vi "IntegerSynByteArrayBulk.vi"(0 "Mode":T1(ring)=enum."Heterodyne", 7 "Input  F1 array":dbl[](array[numeric]), 8 "Clock multiplier":i32=64, 9 "Local Oscillator (IF,f2)":dbl, 10 "f (f1)":i32, 11 "Phase (degrees)":dbl=90.0) -> (3 "output array":u8[](array[numeric]) format="%08b")   [LabVIEW 2015]
panel:
  out "phase":u8 format="%08b"
  # "Heterodyne"
  # "IOtech      Synth           NatInstBrd\n              function          J7          P3                   P1\n              syn1 w clk       A0           3             P0.0  1\n              syn1 D7           A1           5             P0.1  3\n              syn2 w clk       A2           7             PO.2  5\n              syn2 D7           A3           9             PO.3  7\n              syn3 w clk       A4           4             PO.4  9\n              syn3 D7           A5           6             P0.5   11\n              syn1,2 FQ_UD  A6           8             PO.6   13\n              syn3 FQ_UD     A7          10            PO.7   15\n\n              Reset 1,2,3     B4          14             PFI3   23\n\n              SCLK              B0           13            PFI 0  17\n              SYNC              B1           15            PFI 1  19\n              DIN                B2           17             PFI 2  21"
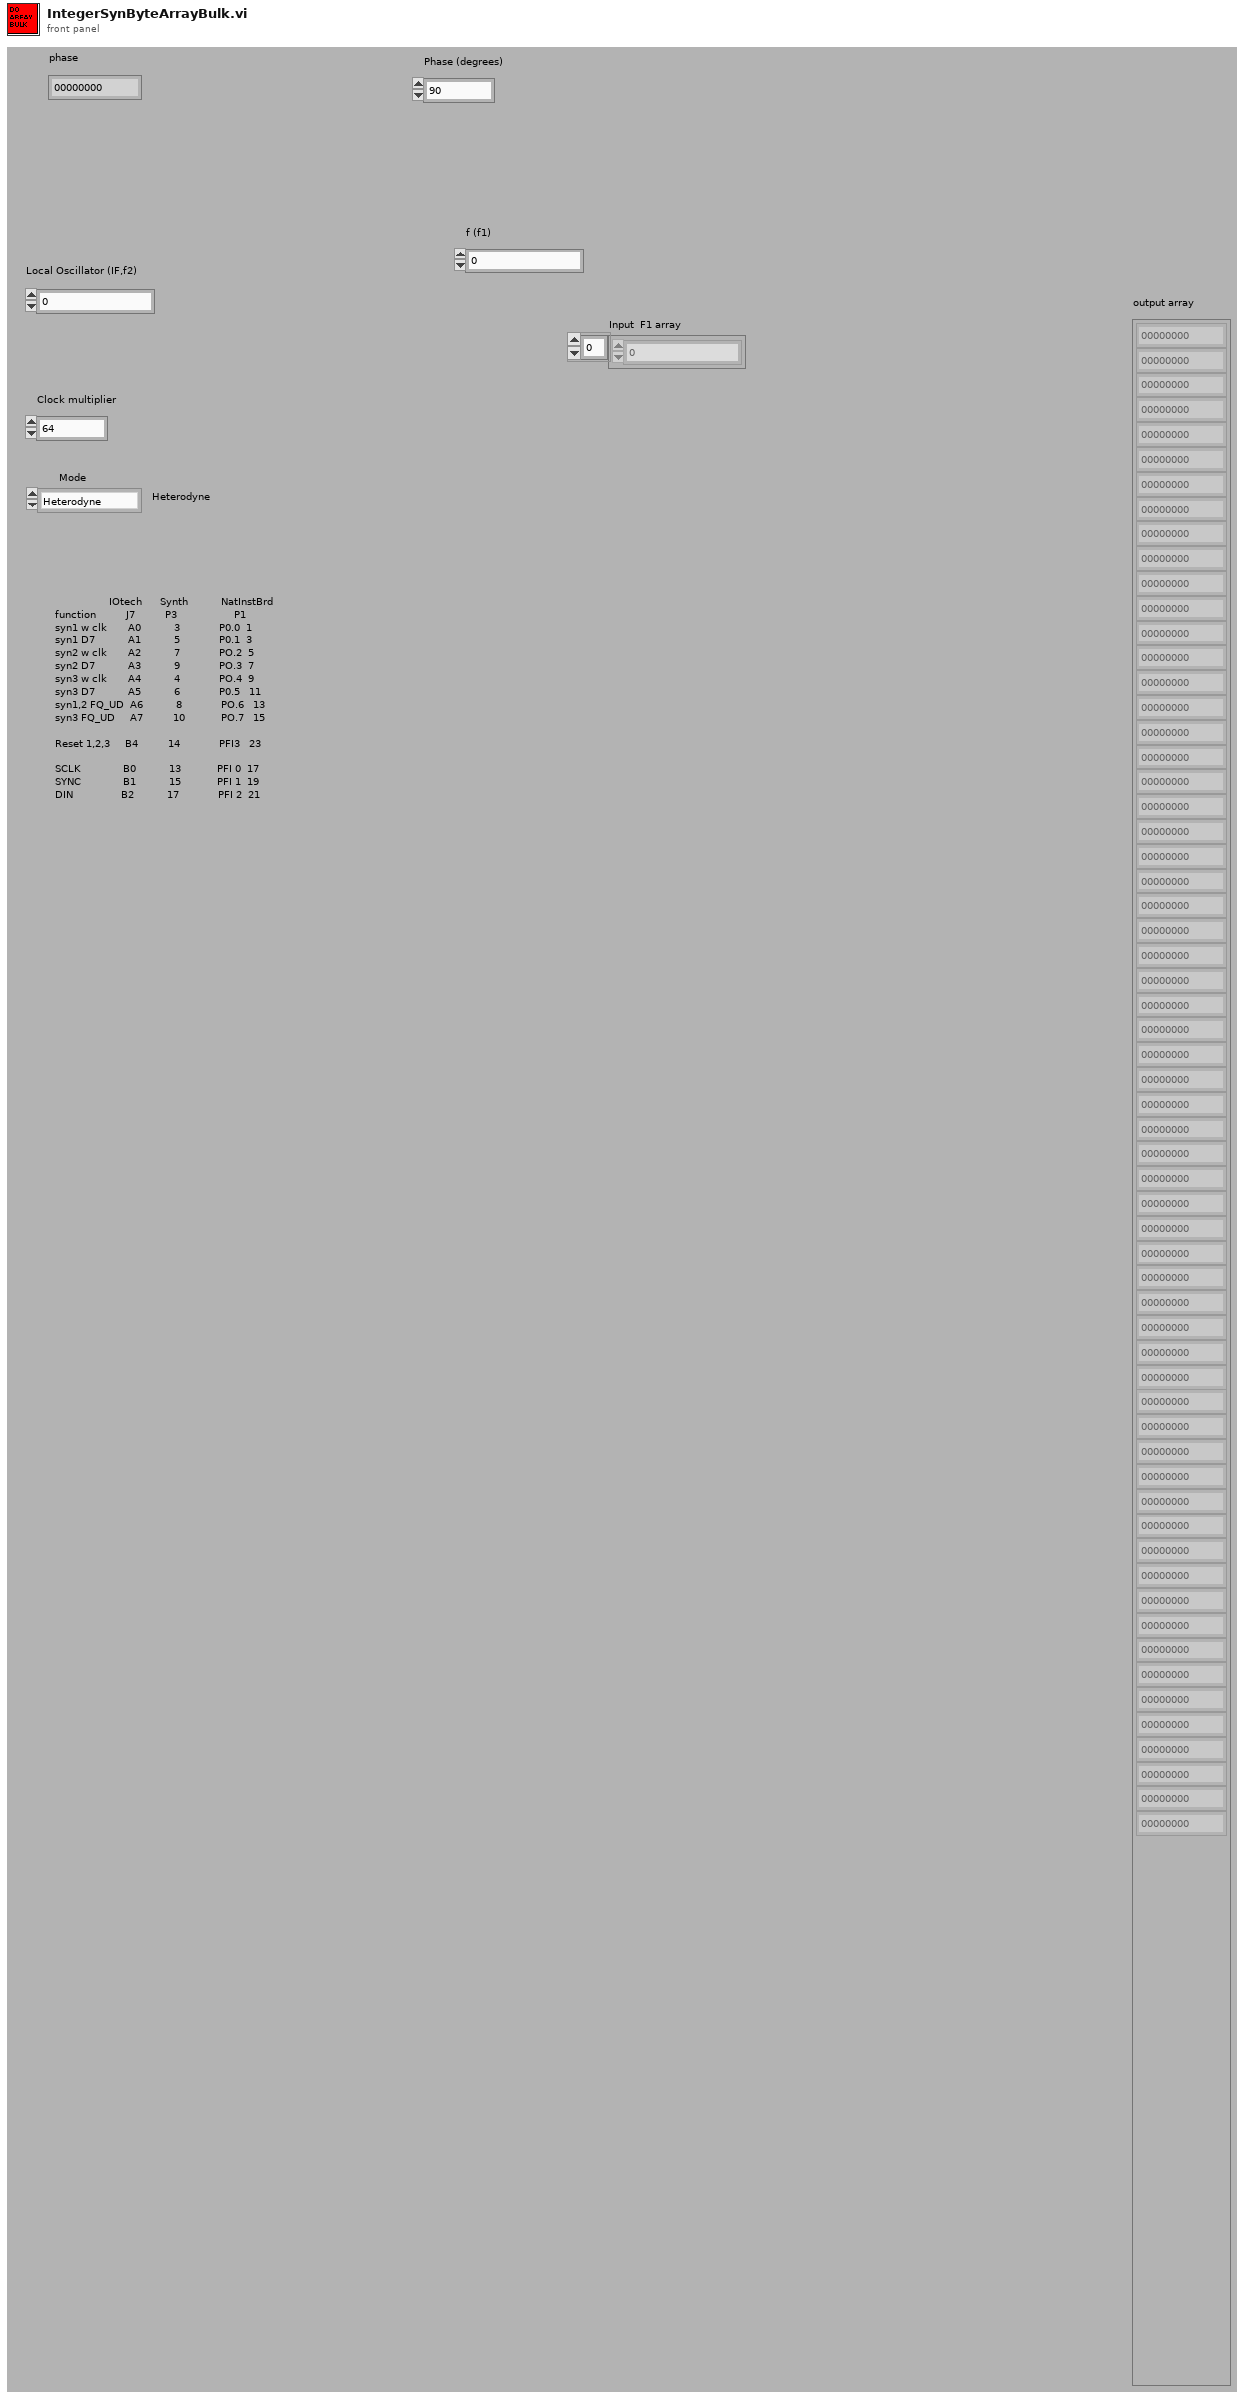
[diagram p1: front panel]
types:
  T1 = enum16{"Direct, clock*f1", "Direct, clock*f2", "Heterodyne"}
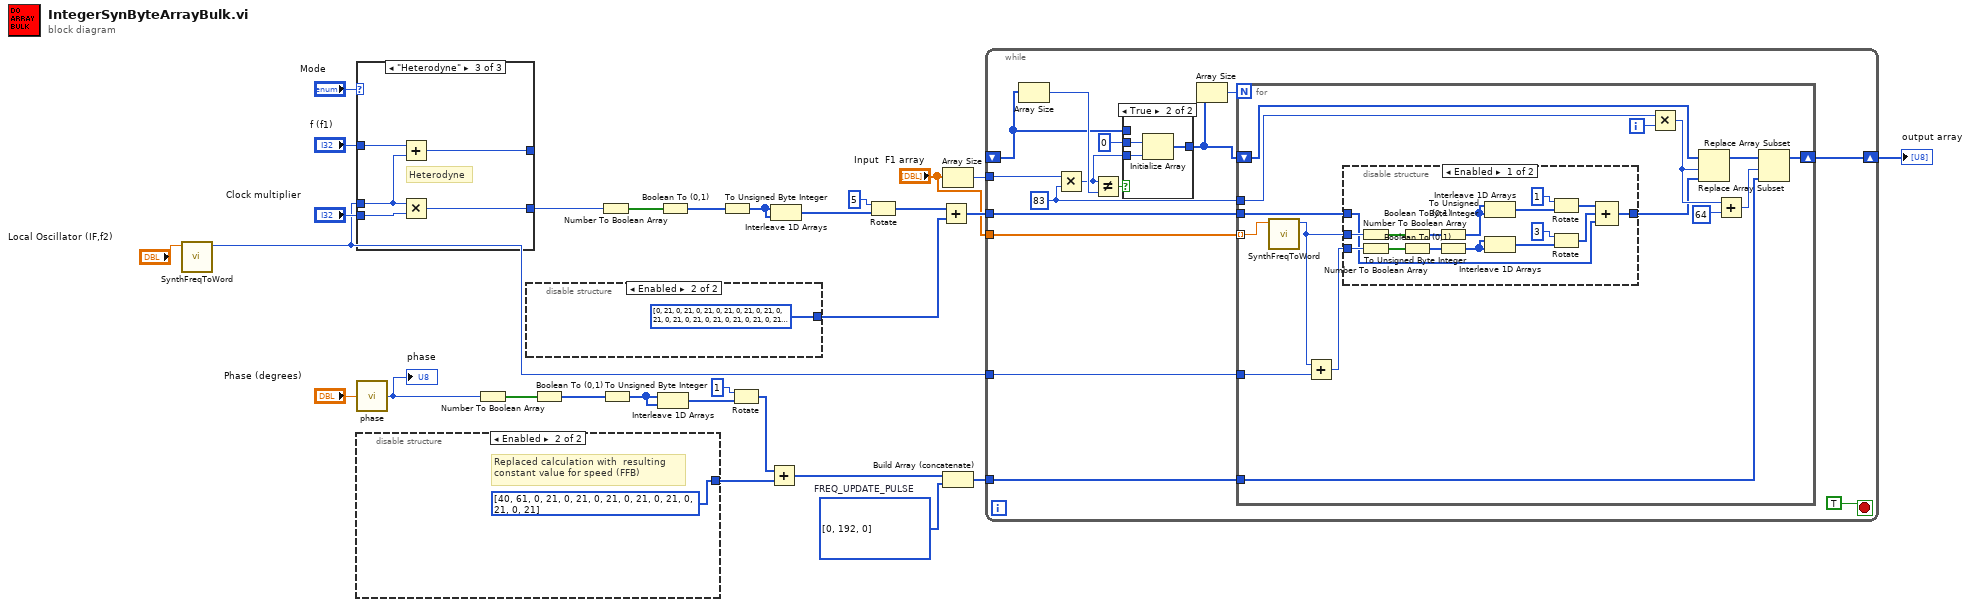
[diagram p0: block diagram]
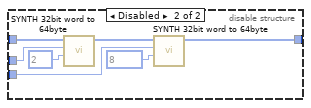
[diagram p3: hidden frame]
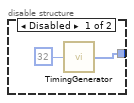
[diagram p4: hidden frame]
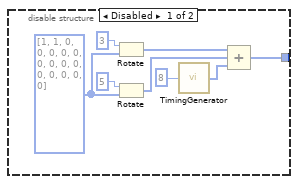
[diagram p5: hidden frame]
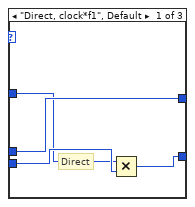
[diagram p6: hidden frame]
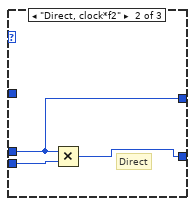
[diagram p7: hidden frame]
diagram:
  w3 = u8[] [0, 192, 0]  # FREQ_UPDATE_PULSE
  n1 = call "SynthFreqToWord.vi"("Frequency (Hz)"="Local Oscillator (IF,f2)") -> ("f-word out"=w5:u32)  [unwired: 8 in, 2 out]
  n2 = case shown="\"Heterodyne\"" "Mode" {
    tunnel: w5 -> [w31 w34 w39]
    tunnel: [w33 w36 w41] -> w24
    tunnel: "Clock multiplier" -> [w32 w35 w40]
    tunnel: [w31 w34 w37] -> _
    tunnel: "f (f1)" -> [w30 _ w38]
    frame "Direct, clock*f1", Default {
      # "Direct"
      n3 = Multiply(x=w30, y=w32) -> (x*y=w33:i32)
    }
    frame "Direct, clock*f2" {
      # "Direct"
      n4 = Multiply(x=w34, y=w35) -> (x*y=w36:u32)
    }
    frame "Heterodyne" {
      # "Heterodyne"
      n5 = Add(x=w38, y=w39) -> (x+y=w37:u32)
      n6 = Multiply(x=w39, y=w40) -> (x*y=w41:u32)
    }
  }
  n7 = call "phase.vi"("Phase"="Phase (degrees)") -> ("Phase Byte"=w18:u8)
  "phase" <- w18
  n8 = disable-structure shown="Enabled" {
    disable-tunnel: [w42 u8[] [40, 61, 0, 21, 0, 21, 0, 21, 0, 21, 0, 21, 0, 21, 0, 21] ("result")] -> w13
    frame Disabled {
      w44 = u8[] [1, 1, 0, 0, 0, 0, 0, 0, 0, 0, 0, 0, 0, 0, 0, 0] ("value")
      n9 = Rotate(1:w44, 2:i8 3) -> (0:w46:u8[])
      n10 = Rotate(1:w44, 2:i8 5) -> (0:w45:u8[])
      n11 = call "TimingGenerator.vi"("Clk String Lngth"=i8 8) -> ("TimingClock"=w43:u8[])
      n12 = Compound Arithmetic op=ADD(w46, w45, w43) -> (w42:u8[])
    }
    frame Enabled {
      # "Replaced calculation with  resulting \nconstant value for speed (FFB)"
    }
  }
  n13 = Number To Boolean Array(number=w18) -> (Boolean array=w21:bool[])
  n14 = disable-structure shown="Enabled" {
    disable-tunnel: [w51 u8[] [0, 21, 0, 21, 0, 21, 0, 21, 0, 21, 0, 21, 0, 21, 0, 21, 0, 21, 0, 21, 0, 21, 0, 21, 0, 21, 0, 21, 0, 21, 0, 21, 0, 21, 0, 21, 0, 21, 0, 21, 0, 21, 0, 21, 0, 21, 0, 21, 0, 21, 0, 21, 0, 21, 0, 21, 0, 21, 0, 21, 0, 21, 0, 21] ("TimingClock")] -> w7
    frame Disabled {
      n15 = call "TimingGenerator.vi"("Clk String Lngth"=i8 32) -> ("TimingClock"=w51:u8[])
    }
    frame Enabled {
    }
  }
  n16 = Boolean To (0,1)(Boolean=w21) -> (0, 1=w20:i16[])
  n17 = Number To Boolean Array(number=w24) -> (Boolean array=w28:bool[])
  n18 = To Unsigned Byte Integer(number=w20) -> (unsigned 8bit integer=w17:u8[])
  n19 = Interleave 1D Arrays(w17, w17) -> (w19:u8[])
  n20 = Boolean To (0,1)(Boolean=w28) -> (0, 1=w27:i16[])
  n21 = To Unsigned Byte Integer(number=w27) -> (unsigned 8bit integer=w22:u8[])
  n22 = Rotate(1:w19, 2:1) -> (0:w12:u8[])
  n23 = Add(x=w12, y=w13) -> (x+y=w9:u8[])
  n24 = Interleave 1D Arrays(w22, w22) -> (w26:u8[])
  n25 = Rotate(1:w26, 2:i8 5) -> (0:w11:u8[])
  n26 = Add(x=w11, y=w7) -> (x+y=w10:u8[])
  n27 = Array Size(array="Input  F1 array") -> (size(s)=w2:i32)
  n28 = Build Array (concatenate)(w9, w3) -> (w4:u8[])
  n29 = while {
    tunnel: w10 -> [w68]
    tunnel: w5 -> [w66]
    tunnel: w4 -> [w65]
    shift-right: [w67] -> w8
    shift-left: _ -> [w58]
    tunnel: w2 -> [w64]
    tunnel: "Input  F1 array" -> [w57]
    stop <- TRUE stop-if-true
    w63 = 83
    n30 = Array Size(array=w58) -> (size(s)=w62:i32)
    n31 = Multiply(x=w64, y=w63) -> (x*y=w60:i32)
    n32 = Not Equal?(x=w60, y=w62) -> (x != y?=w61:bool)
    n33 = case shown="True" w61 {
      tunnel: w60 -> [_ w72]
      tunnel: u8 0 -> [_ w71]
      tunnel: [w69 w70] -> w55
      tunnel: w58 -> [w69 _]
      frame False {
      }
      frame True {
        n34 = Initialize Array(w71, w72) -> (w70:u8[])
      }
    }
    n35 = Array Size(array=w55) -> (size(s)=w54:i32)
    n36 = for {
      N: w54 -> [_]
      shift-right: [w83] -> w67
      shift-left: w55 -> [w87]
      tunnel: w63 -> [w85]
      tunnel: w66 -> [w78]
      tunnel: w68 -> [w74]
      tunnel: w65 -> [w79]
      tunnel: w57 -> [w75] mode=indexing
      i -> [w86]
      n37 = call "SynthFreqToWord.vi"("Frequency (Hz)"=w75) -> ("f-word out"=w76:u32)  [unwired: 8 in, 2 out]
      n38 = Add(x=w76, y=w78) -> (x+y=w77:u32)
      n39 = disable-structure shown="Enabled" {
        disable-tunnel: w76 -> [w95 w110]
        disable-tunnel: w77 -> [w94 w108]
        disable-tunnel: w74 -> [w89 w106]
        disable-tunnel: [w88 w104] -> w73
        frame Enabled {
          n40 = Number To Boolean Array(number=w95) -> (Boolean array=w101:bool[])
          n41 = Number To Boolean Array(number=w94) -> (Boolean array=w103:bool[])
          n42 = Boolean To (0,1)(Boolean=w101) -> (0, 1=w100:i16[])
          n43 = Boolean To (0,1)(Boolean=w103) -> (0, 1=w102:i16[])
          n44 = To Unsigned Byte Integer(number=w100) -> (unsigned 8bit integer=w97:u8[])
          n45 = To Unsigned Byte Integer(number=w102) -> (unsigned 8bit integer=w96:u8[])
          n46 = Interleave 1D Arrays(w97, w97) -> (w99:u8[])
          n47 = Interleave 1D Arrays(w96, w96) -> (w98:u8[])
          n48 = Rotate(1:w99, 2:i8 1) -> (0:w91:u8[])
          n49 = Rotate(1:w98, 2:i8 3) -> (0:w90:u8[])
          n50 = Compound Arithmetic op=ADD(w91, w90, w89) -> (w88:u8[])
        }
        frame Disabled {
          n51 = call "SYNTH 32bit word to 64byte.vi"("Byte to insert"=u8 2, "Freq Word"=w110, "array"=w106) -> ("output array"=w105:u8[])  [unwired: 8 in]
          n52 = call "SYNTH 32bit word to 64byte.vi"("Byte to insert"=u8 8, "Freq Word"=w108, "array"=w105) -> ("output array"=w104:u8[])  [unwired: 8 in]
        }
      }
      n53 = Multiply(x=w85, y=w86) -> (x*y=w82:i32)
      n54 = Replace Array Subset(array=w87, new element=w73, index=w82) -> (w84:u8[])
      n55 = Add(x=w82, y=64) -> (x+y=w80:i32)
      n56 = Replace Array Subset(array=w84, new element=w79, index=w80) -> (w83:u8[])
    }
  }
  "output array" <- w8
